vi "Initialize.vi"(8 "error in (no error)":errorcluster, 11 "Laser in":refnum<class "Laser.lvclass">) -> (0 "error out":errorcluster, 3 "Laser out":refnum<class "Laser.lvclass">)   [LabVIEW 2020, in "Laser.lvlib" / "Laser.lvclass"]
uses:
  Laser.lvclass
  Device/Device/Device.lvclass
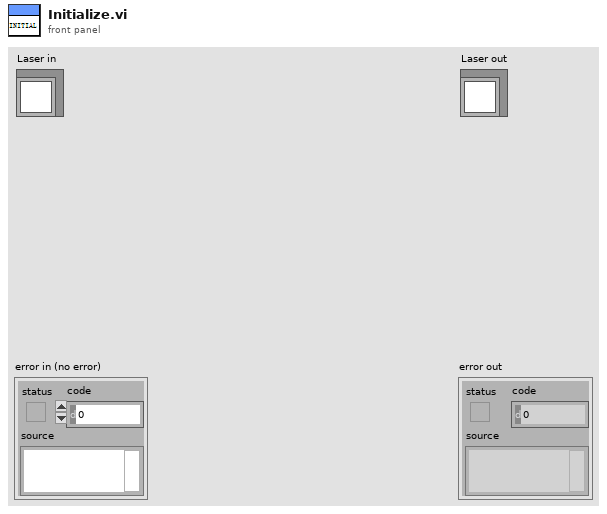
[diagram p1: front panel]
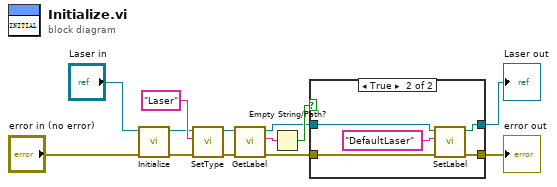
[diagram p0: block diagram]
diagram:
  n1 = call-parent "Initialize.vi"("error in (no error)"="error in (no error)", "GRMActor in"="Laser in") -> ("error out"=w4:errorcluster, "GRMActor out"=w3:refnum<class "Laser.lvclass">)  [unwired: 8 in]
  n2 = call-dynamic "SetType.vi"("error in (no error)"=w4, "Type"="Laser", "GRMActor in"=w3) -> ("error out"=w11:errorcluster, "GRMActor out"=w9:refnum<class "Laser.lvclass">)  [unwired: 7 in]
  n3 = call-dynamic "GetLabel.vi"("error in (no error)"=w11, "GRMActor in"=w9) -> ("error out"=w5:errorcluster, "Label"=w8:string, "GRMActor out"=w6:refnum<class "Laser.lvclass">)  [unwired: 7 in]
  n4 = Empty String/Path?(string/path=w8) -> (empty?=w7:bool)
  n5 = case shown="True" w7 {
    tunnel: w6 -> [w15 w18]
    tunnel: w5 -> [w14 w20]
    tunnel: [w15 w17] -> w2
    tunnel: [w14 w19] -> w1
    frame False {
    }
    frame True {
      n6 = call-dynamic "SetLabel.vi"("error in (no error)"=w20, "Label"="DefaultLaser", "GRMActor in"=w18) -> ("error out"=w19:errorcluster, "GRMActor out"=w17:refnum<class "Laser.lvclass">)  [unwired: 7 in]
    }
  }
  "error out" <- w1
  "Laser out" <- w2
